vi "TCP-Ubidots.vi"() -> ()   [LabVIEW 2020]
uses:
  <vilib>/Instr/_visa.llb/VISA Configure Serial Port (Instr).vi
panel:
  out "adc-dspic33fj32mc202":dbl[](array[slide]) scale=0.0..4095.0
  in  "Baudige (9600)":u32=9600
  in  "puerto":refnum<visa-resource-name>
  in  "stop":bool
  out "concatenated string":string
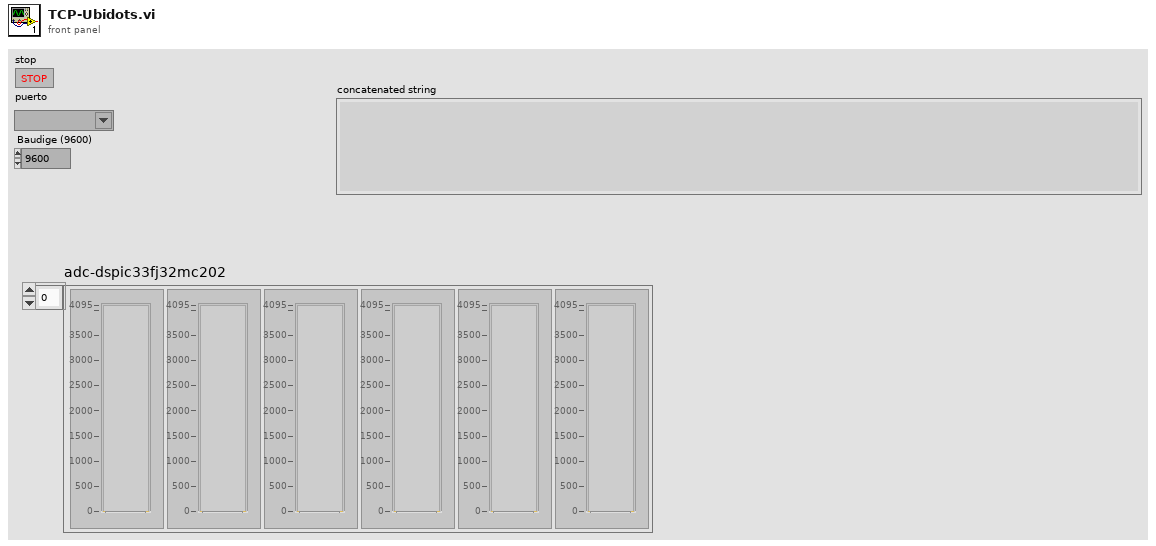
[diagram p1: front panel]
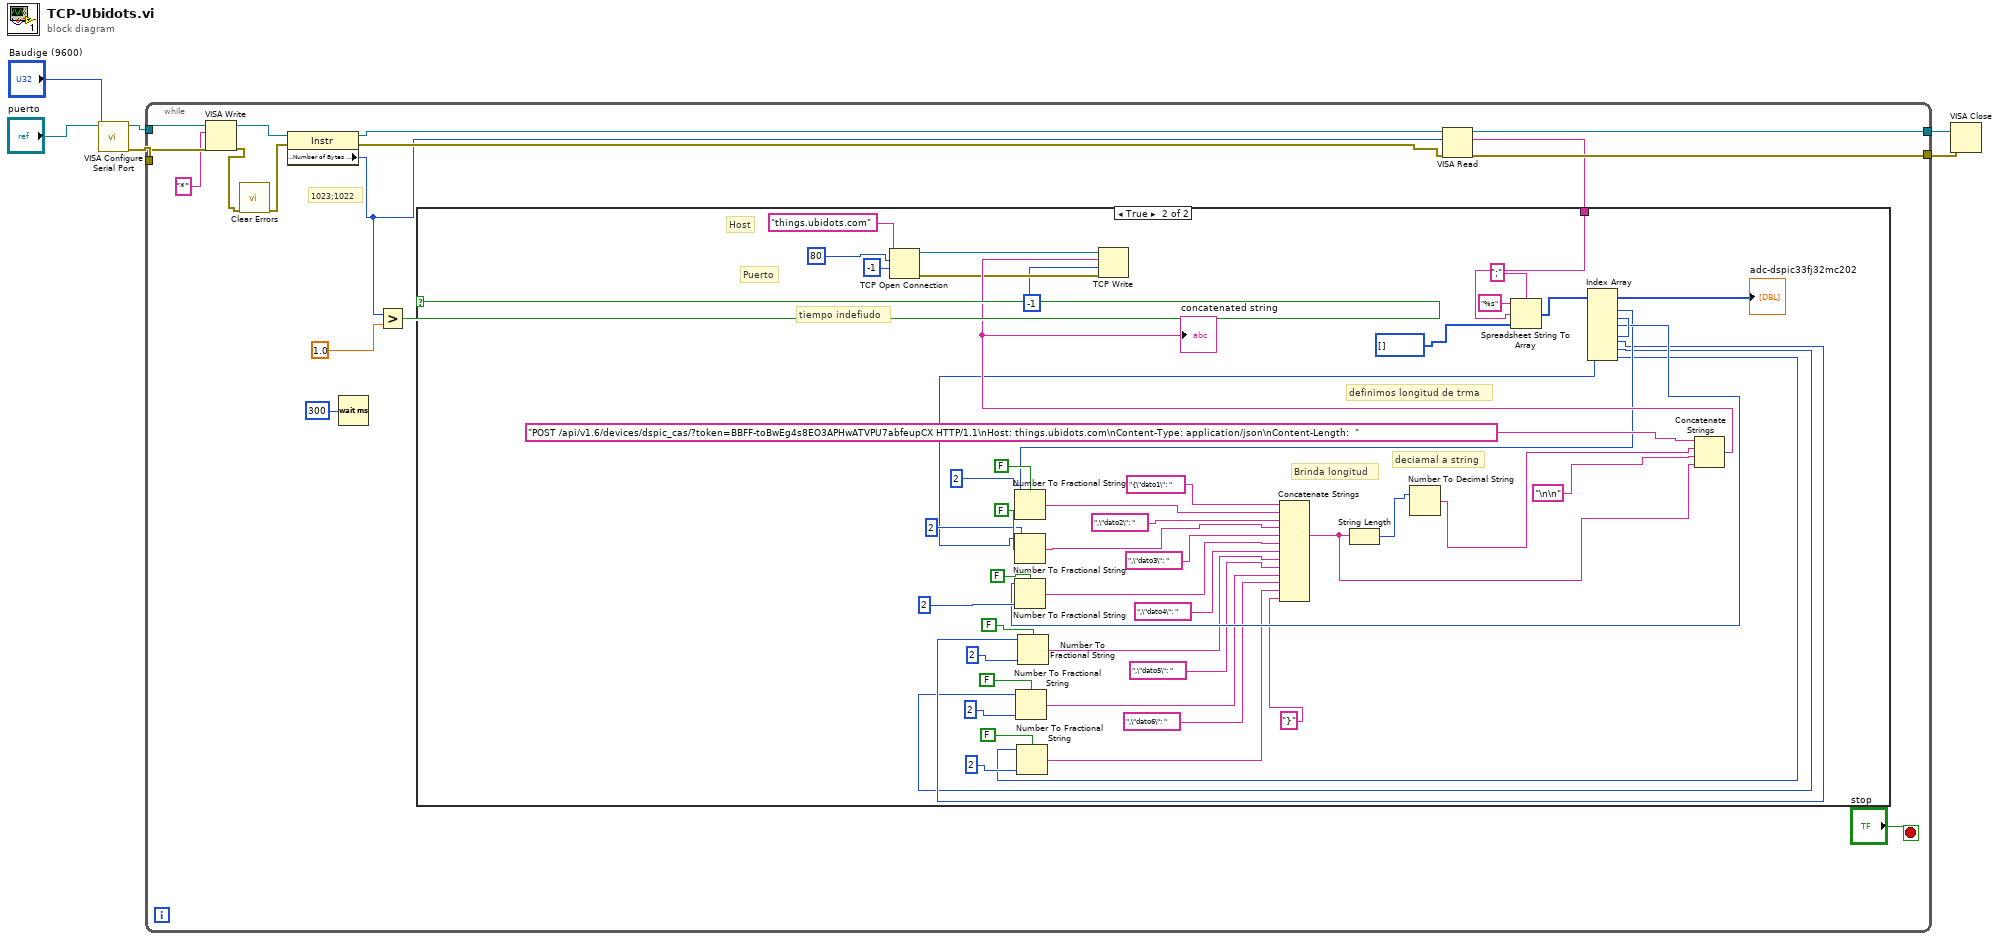
[diagram p0: block diagram]
diagram:
  n1 = call-poly "VISA Configure Serial Port"("VISA resource name"="puerto", "baud rate (9600)"="Baudige (9600)") -> ("VISA resource name out"=w6:refnum<visa-resource-name>, "error out"=w4:errorcluster)  [unwired: 12 in]
  n2 = while {
    tunnel: w6 -> [w11]
    tunnel: [w21] -> w5
    tunnel: w4 -> [w10]
    tunnel: [w19] -> w3
    stop <- "stop" stop-if-true
    # "1023;1022"
    n3 = VISA Write(VISA resource name=w11, write buffer="*", error in (no error)=w10) -> (VISA resource name out=w12:refnum<visa-resource-name>, error out=w8:errorcluster)  [unwired: 1 out]
    n4 = call <vilib>:"Clear Errors.vi"("error in (no error)"=w8) -> ("error out"=w7:errorcluster)  [unwired: 5 in, 1 out]
    n5 = property class="Instr"(reference=w12, error in=w7) -> (reference out=w22:refnum<visa-resource-name>, error out=w20:errorcluster, "Serial Settings:Number of Bytes at Serial Port"=w13:u32)
    n6 = Wait (ms)(milliseconds to wait=u32 300) -> ()  [unwired: 1 out]
    n7 = Greater?(x=w13, y=1.0) -> (0:w14:bool)
    n8 = VISA Read(VISA resource name=w22, byte count=w13, error in (no error)=w20) -> (VISA resource name out=w21:refnum<visa-resource-name>, read buffer=w17:string, error out=w19:errorcluster)  [unwired: 1 out]
    n9 = case shown="True" w14 {
      tunnel: w17 -> [_ w69]
      frame False {
      }
      frame True {
        # "deciamal a string"
        # "Brinda longitud"
        # "definimos longitud de trma"
        # "tiempo indefiudo"
        # "Puerto"
        # "Host"
        n10 = TCP Open Connection(address="things.ubidots.com", remote port or service name=u16 80, timeout ms (60000)=-1) -> (connection ID=w60:refnum<k5>, error out=w61:errorcluster)  [unwired: 2 in]
        n11 = Spreadsheet String To Array(delimiter (Tab)=";", format string="%s", spreadsheet string=w69, array type (2D Dbl)=i32[] []) -> (array=w67:i32[])
        "adc-dspic33fj32mc202" <- w67
        n12 = Index Array(array=w67) -> (element #1=w39:i32, element #2=w41:i32, element #3=w40:i32, element #5=w27:i32, element #6=w26:i32, element #7=w25:i32)  [unwired: 7 in, 1 out]
        n13 = Number To Fractional String(use system decimal point (T)=FALSE, number=w39, precision (6)=i16 2) -> (F-format string=w63:string)  [unwired: 1 in]
        n14 = Number To Fractional String(use system decimal point (T)=FALSE, number=w41, precision (6)=i16 2) -> (F-format string=w64:string)  [unwired: 1 in]
        n15 = Number To Fractional String(use system decimal point (T)=FALSE, number=w40, precision (6)=i16 2) -> (F-format string=w65:string)  [unwired: 1 in]
        n16 = Number To Fractional String(use system decimal point (T)=FALSE, number=w26, precision (6)=i16 2) -> (F-format string=w31:string)  [unwired: 1 in]
        n17 = Number To Fractional String(use system decimal point (T)=FALSE, number=w25, precision (6)=i16 2) -> (F-format string=w29:string)  [unwired: 1 in]
        n18 = Number To Fractional String(use system decimal point (T)=FALSE, number=w27, precision (6)=i16 2) -> (F-format string=w33:string)  [unwired: 1 in]
        n19 = Concatenate Strings("{\"dato1\": " ("string"), w63, ",\"dato2\": " ("string"), w64, ",\"dato3\": " ("string"), w65, ",\"dato4\": " ("string"), w33, ",\"dato5\": " ("string"), w31, ",\"dato6\": " ("string"), w29, "}" ("string")) -> (w66:string)
        n20 = String Length(string=w66) -> (length=w43:i32)
        n21 = Number To Decimal String(number=w43) -> (decimal integer string=w44:string)  [unwired: 1 in]
        n22 = Concatenate Strings("POST /api/v1.6/devices/dspic_cas/?token=BBFF-toBwEg4s8EO3APHwATVPU7abfeupCX HTTP/1.1\nHost: things.ubidots.com\nContent-Type: application/json\nContent-Length:  " ("string"), w44, "\n\n" ("string"), w66) -> (w62:string)
        "concatenated string" <- w62
        n23 = TCP Write(connection ID=w60, data in=w62, error in (no error)=w61, 9:-1 ("timeout ms (25000)")) -> ()  [unwired: 3 out]
      }
    }
  }
  n24 = VISA Close(VISA resource name=w5, error in (no error)=w3) -> ()  [unwired: 1 out]
